vi "Loop_SM.vi"() -> ()   [LabVIEW 2017]
uses:
  ENUM_SM_State.ctl
  ENUM_SM_Action.ctl
  TypeDef/CLUSTER_CMD_WC_Drive.ctl
  TypeDef/ENUM_WC_Drive_DriveMode.ctl
  TypeDef/CLUSTER_Drive_ACT Loop_VBus Data.ctl
  TypeDef/CLUSTER_X and Y.ctl
  TypeDef/CLUSTER_Drive_ACT Loop_Profile Data.ctl
  TypeDef/CLUSTER_Left and Right.ctl
  TypeDef/ENUM_Drive_ACT Loop_Mode.ctl
  TypeDef/CLUSTER_Drive_HW_SRX_Status.ctl
  TypeDef/CLUSTER_4296_SRX_Status.ctl
  TypeDef/CLUSTER_SRX_Status Data.ctl
  TypeDef/CLUSTER_SRX_Encoder Data.ctl
  TypeDef/CLUSTER_SRX_PWM Data.ctl
  TypeDef/CLUSTER_SRX_Analog Data.ctl
  TypeDef/CLUSTER_SRX_Limit Switch Data.ctl
  TypeDef/CLUSTER_SRX_Profile Data.ctl
  TypeDef/CLUST_Targeting Data.ctl
  TypeDef/CLUST_Cube Data.ctl
  TypeDef/CLUST_Road Navigation Data.ctl
  <vilib>/Rock Robotics/WPI/ThirdParty/Sensors/navX/_TypeDefs/FRIC_navX_DeviceNumbersTypeDef.ctl
  _SHARE ALL/Global Share All/Global_STOP.vi
  Globals/Global_CMD_Drive.vi
  Global_ACT Write_Data Out.vi
  Globals/Global_Vision_Data.vi
  Globals/Global_CMD_Gear.vi
  Globals/Global_Drive_Turn_sens.vi
  <vilib>/addons/control/pid/pid.llb/PID (DBL).vi
  Global_SM Write_Data Out.vi
  <vilib>/addons/control/pid/NI_PID_pid.lvlib
  VisionHW Folder/VisionHW.lvlib
panel:
  in  "PID gains Road Follow":T1={"proportional gain (Kc)"=0.01, "integral time (Ti, min)"=0.0, "derivative time (Td, min)"=0.0} {"derivative time (Td, min)" format="%.3f"; "integral time (Ti, min)" format="%.8f"; "proportional gain (Kc)" format="%.8f"}
  in  "PID gains Cube Follow":T1={"proportional gain (Kc)"=0.0015, "integral time (Ti, min)"=0.0, "derivative time (Td, min)"=0.0} {"derivative time (Td, min)" format="%.3f"; "integral time (Ti, min)" format="%.8f"; "proportional gain (Kc)" format="%.8f"}
  in  "Degree allowence":dbl=2.0 format="%#_13g"
  in  "PID gains Lock Angle":T1={"proportional gain (Kc)"=0.01, "integral time (Ti, min)"=0.0, "derivative time (Td, min)"=0.0} {"derivative time (Td, min)" format="%.3f"; "integral time (Ti, min)" format="%.3f"; "proportional gain (Kc)" format="%.8f"}
  in  "Max RPM":dbl=10000.0
  out "Cycle Time (S)":dbl format="%.3g"
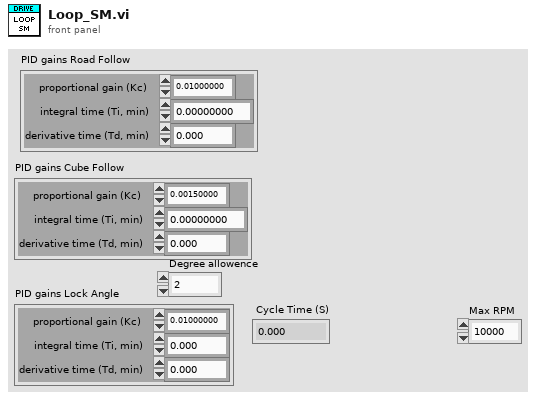
[diagram p1: front panel]
types:
  T1 = cluster{"proportional gain (Kc)":dbl, "integral time (Ti, min)":dbl, "derivative time (Td, min)":dbl}
  T2 = typedef "VisionHW.lvlib/CLUST_Targeting Data.ctl" = cluster{"Cube ":T3, "Road Navigation Data":T4}
  T3 = typedef "VisionHW.lvlib/CLUST_Cube Data.ctl" = cluster{"Height":dbl, "Width":dbl, "Ratio":dbl, "x":i32, "y":i32, "Distance ":i32, "Data Age":dbl}
  T4 = typedef "VisionHW.lvlib/CLUST_Road Navigation Data.ctl" = cluster{"Error":i32, "Data Age":dbl}
  T5 = cluster{"Rollover":dbl, "Yaw":dbl, "Cont Yaw":dbl}
  T6 = typedef "CLUSTER_Drive_HW_SRX_Status.ctl" = cluster{"Rear Left":T7, "Rear Right":T7, "Front Left":T7, "Front Right":T7}
  T7 = typedef "CLUSTER_4296_SRX_Status.ctl" = cluster{"Status":T8, "Encoder":T9, "PWM ":T10, "Analog":T11, "Limit Switches":T12, "Profile":T13}
  T8 = typedef "CLUSTER_SRX_Status Data.ctl" = cluster{"Module Enabled":bool, "Current Profile Slot Select":dbl, "Brake is Enabled":bool, "Applied Throttle":dbl, "Current":dbl, "Battery Voltage":dbl, "Sticky Fault - Under Voltage":bool, "Temperature (C)":dbl, "Sticky Fault - Over Temp":bool, "CAN Error":errorcluster, "Control 5 Is Supported":bool}
  T9 = typedef "CLUSTER_SRX_Encoder Data.ctl" = cluster{"Closed Loop Error":dbl, "Sensor Position":dbl, "Sensor Velocity":dbl, "Encoder Position":dbl, "Encoder Velocity":dbl, "Encoder Index Count":dbl, "Encoder A Pin State":bool, "Encoder B Pin State":bool, "Encoder Index Pin State":bool, "Pos Div 8":bool, "Vel Div 4":bool}
  T10 = typedef "CLUSTER_SRX_PWM Data.ctl" = cluster{"Closed Loop Error":dbl, "Pulse Width Position":i32, "Pulse Width Velocity":i32, "Pulse Width Rise To Rise (us)":i32, "Pulse Width Rise To Fall (us)":i32}
  T11 = typedef "CLUSTER_SRX_Analog Data.ctl" = cluster{"Closed Loop Error":dbl, "Analog In":dbl, "Analog In Velocity":dbl}
  T12 = typedef "CLUSTER_SRX_Limit Switch Data.ctl" = cluster{"Forward Limit Switch Closed":bool, "Reverse Limit Switch Closed":bool, "Sticky Fault - Forward Limit":bool, "Sticky Fault - Reverse Limit":bool, "Sticky Fault - Forward Soft Limit":bool, "Sticky Fault - Reverse Soft Limit":bool}
  T13 = typedef "CLUSTER_SRX_Profile Data.ctl" = cluster{"Mot Prof Active Is Under Run":bool, "Mot Prof Active Has Under Run":bool, "Mot Prof Active Is Last":bool, "Mot Prof Active Velocity Only":bool, "Mot Prof Active Is Valid":bool, "Mot Prof Buffer Is Full":bool, "Mot Prof Active Profile Slot Select":i32, "Mot Prof NextID":i32, "Mot Prof Count":i32, "Mot Prof Active Velocity":dbl, "Mot Prof Active Position":dbl, "Mot Prof Output Enable":i32}
  T14 = typedef "ENUM_Drive_ACT Loop_Mode.ctl" = enum16{"Stop", "Position", "VBus", "Profile"}
  T15 = typedef "CLUSTER_Left and Right.ctl" = cluster{"Left":dbl, "Right":dbl}
  T16 = typedef "CLUSTER_CMD_WC_Drive.ctl" = cluster{"Drive_Mode":T17, "VBus":T18, "Profile":T20, "Zero Drive Encoders":bool, "Set Target Position(IN)":dbl, "Target Angle(Degree)":dbl, "Lock Angle":bool, "Zero YAW":bool, "Follow Cubes":bool, "Follow Road":bool}
  T17 = typedef "ENUM_WC_Drive_DriveMode.ctl" = enum16{"Motion Profile", "CrossLineAuto", "VBus", "Stop"}
  T18 = typedef "CLUSTER_Drive_ACT Loop_VBus Data.ctl" = cluster{"Drive":T19, "Turbo":bool}
  T19 = typedef "CLUSTER_X and Y.ctl" = cluster{"Steer":dbl, "Throtle":dbl}
  T20 = typedef "CLUSTER_Drive_ACT Loop_Profile Data.ctl" = cluster{"Start":bool}
  T21 = typedef "ENUM_SM_Action.ctl" = enum16{"No Action", "Reset Time", "Reset All", "Drive", "Zero YAW", "Shift", "Calculate Sensitivity"}
  T22 = typedef "ENUM_SM_State.ctl" = enum16{"Startup", "VBus", "VBus Lock Angle", "Idle", "Road Follow", "Follow Cube", "Shutdown"}
  T23 = cluster{"Action":T21, "State":T22, "Previous State":T22, "Current Time":timestamp, "Previous Time":timestamp, "Start Time":timestamp, "Target Time (ms)":u32, "Cycle Time(S)":dbl, "CMD_Drive":T16, "VBus Output":T15, "Mode Output":T14, "MQuickStopAccumulator":dbl, "SRX_Status":T6, "Sensitivity":dbl, "NavX Yaw":cluster{"Rollover":dbl, "Yaw":dbl, "Cont Yaw":dbl}, "LockAngle":bool, "Zero YAW":bool, "Target Cube Position (Pixels)":dbl, "Follow Cube":bool, "Follow Road":bool, "Targeting Data":T2, "Gear shift":bool, "Max Sensitivity High Gear":dbl, "Max Sensitivity Low Gear":dbl, "Min Sensitivity High Gear":dbl, "Min Sensitivity Low Gear":dbl}
  T24 = typedef "FRIC_navX_DeviceNumbersTypeDef.ctl" = enum16{"Dev0", "Dev1", "Dev2", "Dev3"}
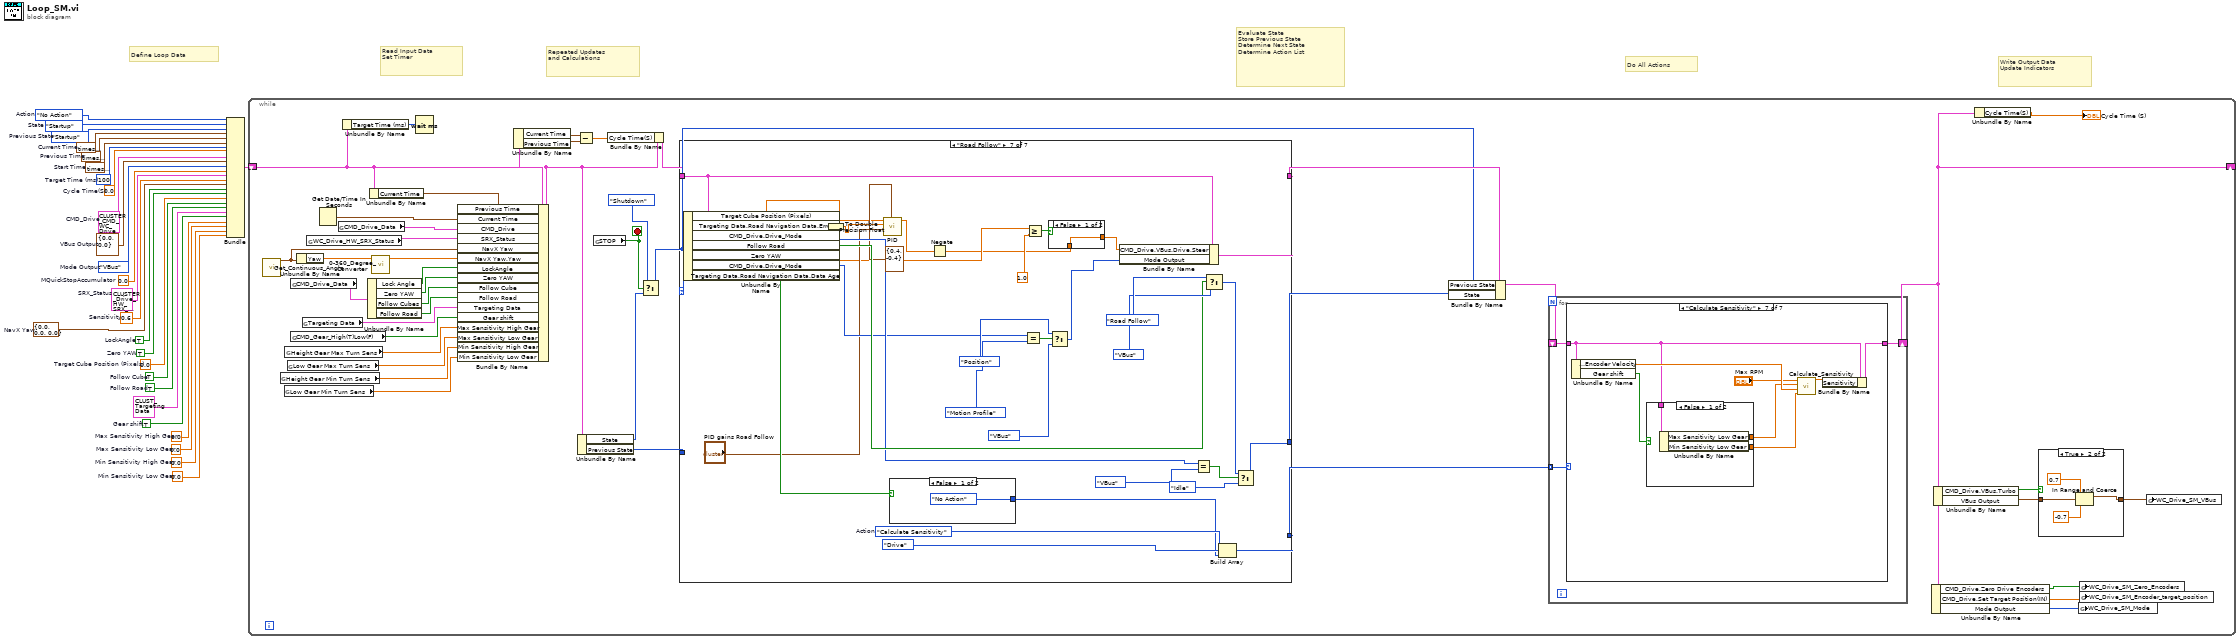
[diagram p0: block diagram]
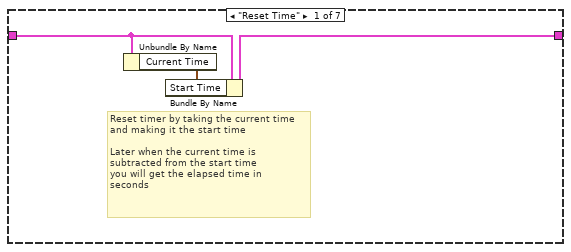
[diagram p3: hidden frame]
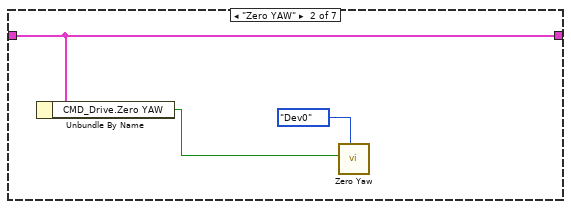
[diagram p4: hidden frame]
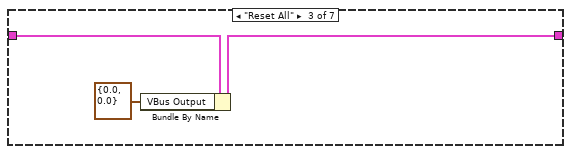
[diagram p5: hidden frame]
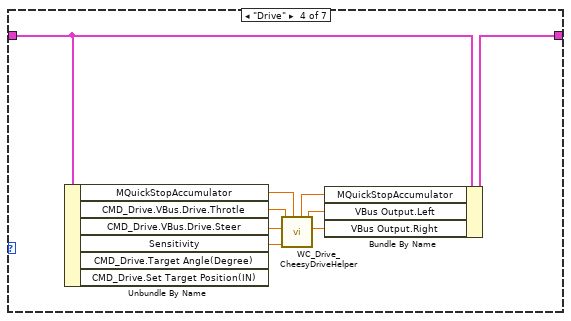
[diagram p6: hidden frame]
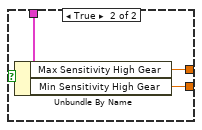
[diagram p9: hidden frame]
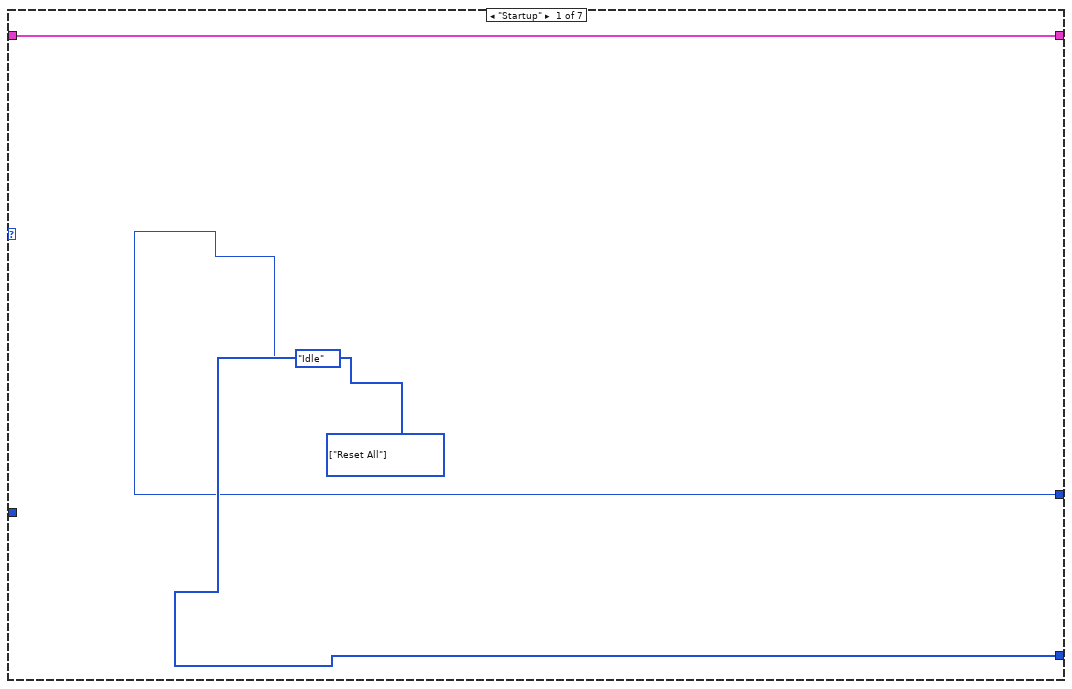
[diagram p10: hidden frame]
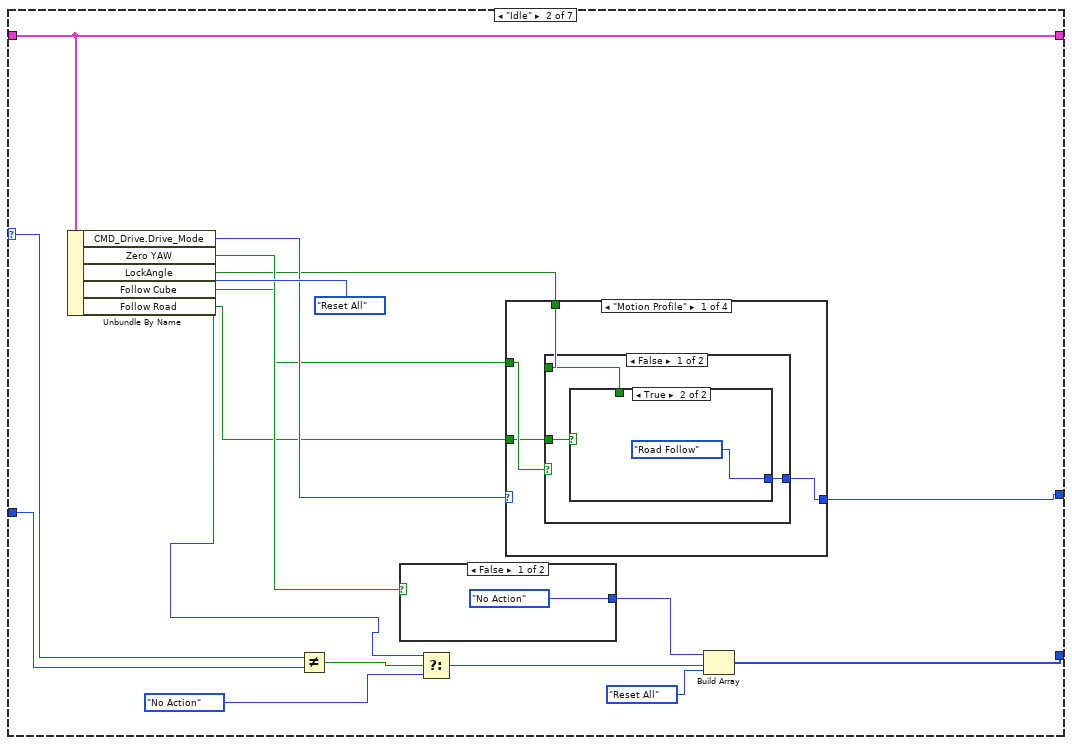
[diagram p11: hidden frame]
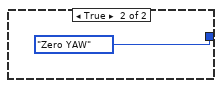
[diagram p12: hidden frame]
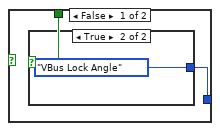
[diagram p13: hidden frame]
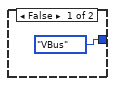
[diagram p14: hidden frame]
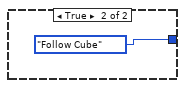
[diagram p15: hidden frame]
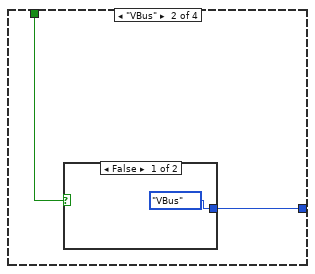
[diagram p16: hidden frame]
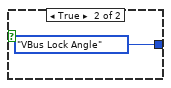
[diagram p17: hidden frame]
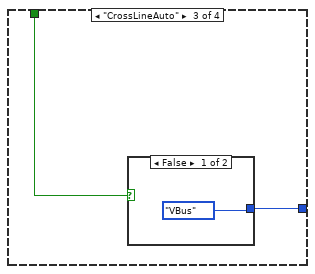
[diagram p18: hidden frame]
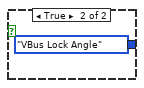
[diagram p19: hidden frame]
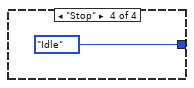
[diagram p20: hidden frame]
diagram:
  w1 = 0.0  # Min Sensitivity Low Gear
  w2 = 0.0  # Min Sensitivity High Gear
  w3 = 0.0  # Max Sensitivity Low Gear
  w4 = 0.0  # Max Sensitivity High Gear
  w5 = TRUE  # Gear shift
  w7 = TRUE  # Follow Road
  w8 = TRUE  # Follow Cube
  w9 = 0.0  # Target Cube Position (Pixels)
  w10 = TRUE  # Zero YAW
  w11 = TRUE  # LockAngle
  w12 = T5 {"Rollover"=0.0, "Yaw"=0.0, "Cont Yaw"=0.0}  # NavX Yaw
  w13 = 0.6  # Sensitivity
  w14 = T6 {"Rear Left"={"Status"={"Module Enabled"=FALSE, "Current Profile Slot Select"=0.0, "Brake is Enabled"=TRUE, "Applied Throttle"=0.0, "Current"=0.0, "Battery Voltage"=12.450000000000001, "Sticky Fault - Under Voltage"=TRUE, "Temperature (C)"=30.645161290322577, "Sticky Fault - Over Temp"=FALSE, "CAN Error"={"status"=FALSE, "code"=0, "source"=""}, "Control 5 Is Supported"=TRUE}, "Encoder"={"Closed Loop Error"=0.0, "Sensor Position"=-847.859619140625, "Sensor Velocity"=0.0, "Encoder Position"=-3472833.0, "Encoder Velocity"=0.0, "Encoder Index Count"=-9452.0, "Encoder A Pin State"=FALSE, "Encoder B Pin State"=FALSE, "Encoder Index Pin State"=FALSE, "Pos Div 8"=FALSE, "Vel Div 4"=FALSE}, "PWM "={"Closed Loop Error"=0.0, "Pulse Width Position"=-3472224, "Pulse Width Velocity"=0, "Pulse Width Rise To Rise (us)"=4187, "Pulse Width Rise To Fall (us)"=1210}, "Analog"={"Closed Loop Error"=0.0, "Analog In"=105.0, "Analog In Velocity"=0.0}, "Limit Switches"={"Forward Limit Switch Closed"=FALSE, "Reverse Limit Switch Closed"=FALSE, "Sticky Fault - Forward Limit"=FALSE, "Sticky Fault - Reverse Limit"=TRUE, "Sticky Fault - Forward Soft Limit"=FALSE, "Sticky Fault - Reverse Soft Limit"=FALSE}, "Profile"={"Mot Prof Active Is Under Run"=FALSE, "Mot Prof Active Has Under Run"=FALSE, "Mot Prof Active Is Last"=FALSE, "Mot Prof Active Velocity Only"=FALSE, "Mot Prof Active Is Valid"=FALSE, "Mot Prof Buffer Is Full"=FALSE, "Mot Prof Active Profile Slot Select"=0, "Mot Prof NextID"=0, "Mot Prof Count"=0, "Mot Prof Active Velocity"=0.0, "Mot Prof Active Position"=0.0, "Mot Prof Output Enable"=0}}, "Rear Right"={"Status"={"Module Enabled"=FALSE, "Current Profile Slot Select"=0.0, "Brake is Enabled"=TRUE, "Applied Throttle"=0.0, "Current"=0.125, "Battery Voltage"=12.4, "Sticky Fault - Under Voltage"=TRUE, "Temperature (C)"=27.41935483870968, "Sticky Fault - Over Temp"=FALSE, "CAN Error"={"status"=FALSE, "code"=0, "source"=""}, "Control 5 Is Supported"=TRUE}, "Encoder"={"Closed Loop Error"=0.0, "Sensor Position"=-228.95263671875, "Sensor Velocity"=0.0, "Encoder Position"=937790.0, "Encoder Velocity"=0.0, "Encoder Index Count"=2928.0, "Encoder A Pin State"=FALSE, "Encoder B Pin State"=TRUE, "Encoder Index Pin State"=TRUE, "Pos Div 8"=FALSE, "Vel Div 4"=FALSE}, "PWM "={"Closed Loop Error"=0.0, "Pulse Width Position"=937817, "Pulse Width Velocity"=0, "Pulse Width Rise To Rise (us)"=4128, "Pulse Width Rise To Fall (us)"=3960}, "Analog"={"Closed Loop Error"=0.0, "Analog In"=103.0, "Analog In Velocity"=0.0}, "Limit Switches"={"Forward Limit Switch Closed"=FALSE, "Reverse Limit Switch Closed"=FALSE, "Sticky Fault - Forward Limit"=FALSE, "Sticky Fault - Reverse Limit"=FALSE, "Sticky Fault - Forward Soft Limit"=FALSE, "Sticky Fault - Reverse Soft Limit"=FALSE}, "Profile"={"Mot Prof Active Is Under Run"=FALSE, "Mot Prof Active Has Under Run"=FALSE, "Mot Prof Active Is Last"=FALSE, "Mot Prof Active Velocity Only"=FALSE, "Mot Prof Active Is Valid"=FALSE, "Mot Prof Buffer Is Full"=FALSE, "Mot Prof Active Profile Slot Select"=0, "Mot Prof NextID"=0, "Mot Prof Count"=0, "Mot Prof Active Velocity"=0.0, "Mot Prof Active Position"=0.0, "Mot Prof Output Enable"=0}}, "Front Left"={"Status"={"Module Enabled"=FALSE, "Current Profile Slot Select"=0.0, "Brake is Enabled"=TRUE, "Applied Throttle"=0.0, "Current"=0.0, "Battery Voltage"=12.4, "Sticky Fault - Under Voltage"=TRUE, "Temperature (C)"=28.709677419354833, "Sticky Fault - Over Temp"=FALSE, "CAN Error"={"status"=FALSE, "code"=0, "source"=""}, "Control 5 Is Supported"=TRUE}, "Encoder"={"Closed Loop Error"=0.0, "Sensor Position"=0.0, "Sensor Velocity"=0.0, "Encoder Position"=0.0, "Encoder Velocity"=0.0, "Encoder Index Count"=0.0, "Encoder A Pin State"=TRUE, "Encoder B Pin State"=TRUE, "Encoder Index Pin State"=TRUE, "Pos Div 8"=FALSE, "Vel Div 4"=FALSE}, "PWM "={"Closed Loop Error"=0.0, "Pulse Width Position"=0, "Pulse Width Velocity"=0, "Pulse Width Rise To Rise (us)"=0, "Pulse Width Rise To Fall (us)"=0}, "Analog"={"Closed Loop Error"=0.0, "Analog In"=105.0, "Analog In Velocity"=0.0}, "Limit Switches"={"Forward Limit Switch Closed"=FALSE, "Reverse Limit Switch Closed"=FALSE, "Sticky Fault - Forward Limit"=FALSE, "Sticky Fault - Reverse Limit"=FALSE, "Sticky Fault - Forward Soft Limit"=FALSE, "Sticky Fault - Reverse Soft Limit"=FALSE}, "Profile"={"Mot Prof Active Is Under Run"=FALSE, "Mot Prof Active Has Under Run"=FALSE, "Mot Prof Active Is Last"=FALSE, "Mot Prof Active Velocity Only"=FALSE, "Mot Prof Active Is Valid"=FALSE, "Mot Prof Buffer Is Full"=FALSE, "Mot Prof Active Profile Slot Select"=0, "Mot Prof NextID"=0, "Mot Prof Count"=0, "Mot Prof Active Velocity"=0.0, "Mot Prof Active Position"=0.0, "Mot Prof Output Enable"=0}}, "Front Right"={"Status"={"Module Enabled"=FALSE, "Current Profile Slot Select"=0.0, "Brake is Enabled"=TRUE, "Applied Throttle"=0.0, "Current"=0.0, "Battery Voltage"=12.35, "Sticky Fault - Under Voltage"=TRUE, "Temperature (C)"=26.77419354838709, "Sticky Fault - Over Temp"=FALSE, "CAN Error"={"status"=FALSE, "code"=0, "source"=""}, "Control 5 Is Supported"=TRUE}, "Encoder"={"Closed Loop Error"=0.0, "Sensor Position"=0.0, "Sensor Velocity"=0.0, "Encoder Position"=0.0, "Encoder Velocity"=0.0, "Encoder Index Count"=0.0, "Encoder A Pin State"=TRUE, "Encoder B Pin State"=TRUE, "Encoder Index Pin State"=TRUE, "Pos Div 8"=FALSE, "Vel Div 4"=FALSE}, "PWM "={"Closed Loop Error"=0.0, "Pulse Width Position"=0, "Pulse Width Velocity"=0, "Pulse Width Rise To Rise (us)"=0, "Pulse Width Rise To Fall (us)"=0}, "Analog"={"Closed Loop Error"=0.0, "Analog In"=102.0, "Analog In Velocity"=0.0}, "Limit Switches"={"Forward Limit Switch Closed"=FALSE, "Reverse Limit Switch Closed"=FALSE, "Sticky Fault - Forward Limit"=FALSE, "Sticky Fault - Reverse Limit"=TRUE, "Sticky Fault - Forward Soft Limit"=FALSE, "Sticky Fault - Reverse Soft Limit"=FALSE}, "Profile"={"Mot Prof Active Is Under Run"=FALSE, "Mot Prof Active Has Under Run"=FALSE, "Mot Prof Active Is Last"=FALSE, "Mot Prof Active Velocity Only"=FALSE, "Mot Prof Active Is Valid"=FALSE, "Mot Prof Buffer Is Full"=FALSE, "Mot Prof Active Profile Slot Select"=0, "Mot Prof NextID"=0, "Mot Prof Count"=0, "Mot Prof Active Velocity"=0.0, "Mot Prof Active Position"=0.0, "Mot Prof Output Enable"=0}}}  # SRX_Status
  w15 = 0.0  # MQuickStopAccumulator
  w16 = ENUM_Drive_ACT_Loop_Mode."VBus"  # Mode Output
  w17 = T15 {"Left"=0.0, "Right"=0.0}  # VBus Output
  w18 = T16 {"Drive_Mode"=enum."Motion Profile", "VBus"={"Drive"={"Steer"=0.0, "Throtle"=0.0}, "Turbo"=FALSE}, "Profile"={"Start"=FALSE}, "Zero Drive Encoders"=FALSE, "Set Target Position(IN)"=0.0, "Target Angle(Degree)"=0.0, "Lock Angle"=FALSE, "Zero YAW"=FALSE, "Follow Cubes"=FALSE, "Follow Road"=FALSE}  # CMD_Drive
  w19 = ENUM_SM_Action."No Action"  # Action
  w20 = 0.0  # Cycle Time(S)
  w21 = ENUM_SM_State."Startup"  # Previous State
  w22 = timestamp(0 s since 1904-01-01)  # Previous Time
  w23 = u32 100  # Target Time (ms)
  w24 = timestamp(0 s since 1904-01-01)  # Start Time
  w25 = timestamp(0 s since 1904-01-01)  # Current Time
  w26 = ENUM_SM_State."Startup"  # State
  # "Define Loop Data"
  # "Repeated Updates\nand Calculations"
  # "Read Input Data\nSet Timer"
  # "Evaluate State\nStore Previous State\nDetermine Next State\nDetermine Action List"
  # "Do All Actions"
  # "Write Output Data\nUpdate Indicators"
  n1 = Bundle("Action"=w19, "State"=w26, "Previous State"=w21, "Current Time"=w25, "Previous Time"=w22, "Start Time"=w24, "Target Time (ms)"=w23, "Cycle Time(S)"=w20, "CMD_Drive"=w18, "VBus Output"=w17, "Mode Output"=w16, "MQuickStopAccumulator"=w15, "SRX_Status"=w14, "Sensitivity"=w13, "NavX Yaw"=w12, "LockAngle"=w11, "Zero YAW"=w10, "Target Cube Position (Pixels)"=w9, "Follow Cube"=w8, "Follow Road"=w7, "Targeting Data"=T2 {"Cube "={"Height"=0.0, "Width"=0.0, "Ratio"=0.0, "x"=0, "y"=0, "Distance "=0, "Data Age"=0.0}, "Road Navigation Data"={"Error"=0, "Data Age"=0.0}}, "Gear shift"=w5, "Max Sensitivity High Gear"=w4, "Max Sensitivity Low Gear"=w3, "Min Sensitivity High Gear"=w2, "Min Sensitivity Low Gear"=w1) -> (w27:T23)  [unwired: 1 in]
  n2 = while {
    shift-right: [w49] -> _
    shift-left: w27 -> [w60]
    stop <- w65 stop-if-true
    n3 = call <vilib>:"Get_Continuous_Angle.vi"() -> ("Continuous Angle"=w45:T5)  [unwired: 11 in]
    n4 = global read "Global_Drive_Turn_sens.vi" "Height Gear Min Turn Sens"() -> (w29:dbl)
    n5 = global read "Global_Drive_Turn_sens.vi" "Low Gear Min Turn Sens"() -> (w28:dbl)
    n6 = global read "Global_Drive_Turn_sens.vi" "Height Gear Max Turn Sens"() -> (w31:dbl)
    n7 = global read "Global_Drive_Turn_sens.vi" "Low Gear Max Turn Sens"() -> (w30:dbl)
    n8 = global read "Global_CMD_Drive.vi" "CMD_Drive_Data"() -> (w40:T16)
    n9 = global read "Global_CMD_Gear.vi" "CMD_Gear_High(T)Low(F)"() -> (w32:bool)
    n10 = Unbundle By Name(w45) -> ("Yaw"=w44:dbl)
    n11 = global read "Global_Vision_Data.vi" "Targeting Data"() -> (w33:T2)
    n12 = global read "Global_ACT Write_Data Out.vi" "WC_Drive_HW_SRX_Status"() -> (w46:T6)
    n13 = Get Date/Time In Seconds() -> (seconds since 1Jan1904=w69:timestamp)
    n14 = global read "Global_CMD_Drive.vi" "CMD_Drive_Data"() -> (w50:T16)
    n15 = Unbundle By Name(w60) -> ("Target Time (ms)"=w62:u32)
    n16 = Unbundle By Name(w40) -> ("Lock Angle"=w39:bool, "Zero YAW"=w38:bool, "Follow Cubes"=w35:bool, "Follow Road"=w34:bool)
    n17 = Unbundle By Name(w60) -> ("Current Time"=w61:timestamp)
    n18 = call "0-360_Degree_Converter.vi"("Yaw in"=w44) -> ("Yaw out"=w41:dbl)  [unwired: 10 in]
    n19 = Wait (ms)(milliseconds to wait=w62) -> ()  [unwired: 1 out]
    n20 = Bundle By Name(cluster=w60, "Previous Time"=w61, "Current Time"=w69, "CMD_Drive"=w50, "SRX_Status"=w46, "NavX Yaw"=w45, "NavX Yaw.Yaw"=w41, "LockAngle"=w39, "Zero YAW"=w38, "Follow Cube"=w35, "Follow Road"=w34, "Targeting Data"=w33, "Gear shift"=w32, "Max Sensitivity High Gear"=w31, "Max Sensitivity Low Gear"=w30, "Min Sensitivity High Gear"=w29, "Min Sensitivity Low Gear"=w28) -> (w42:T23)
    n21 = Unbundle By Name(w42) -> ("Current Time"=w55:timestamp, "Previous Time"=w56:timestamp)
    n22 = Subtract(x=w55, y=w56) -> (x-y=w53:dbl)
    n23 = Unbundle By Name(w42) -> ("State"=w63:T22, "Previous State"=w59:T22)
    n24 = global read "Global_STOP.vi" "STOP"() -> (w65:bool)
    n25 = Bundle By Name(cluster=w42, "Cycle Time(S)"=w53) -> (w54:T23)
    n26 = Select(t=ENUM_SM_State."Shutdown" ("State"), s=w65, f=w63) -> (s? t:f=w58:T22)
    n27 = case shown="\"Road Follow\"" w58 {
      selector: w58 -> [_ w124 _ _ _ _ _]
      tunnel: w54 -> [w114 w130 w159 w188 w213 w248 w285]
      tunnel: [w114 w130 w158 w188 w217 w252 w289] -> w67
      tunnel: [ENUM_SM_State."Idle" ("State") w121 w178 ENUM_SM_State."Shutdown" ("State") w205 w241 w278] -> w66
      tunnel: [w113 w125 w174 w186 w214 w249 w286] -> w52
      tunnel: w59 -> [_ w123 _ _ _ _ _]
      frame "Startup" {
        w113 = T21[] [enum."Reset All"] items=["No Action", "Reset Time", "Reset All", "Drive", "Zero YAW", "Shift", "Calculate Sensitivity"] ("Actions")
      }
      frame "Idle" {
        n28 = Unbundle By Name(w130) -> ("CMD_Drive.Drive_Mode"=w122:T17, "Zero YAW"=w119:bool, "LockAngle"=w118:bool, "Follow Cube"=w116:bool, "Follow Road"=w115:bool)
        n29 = Not Equal?(x=w124, y=w123) -> (x != y?=w129:bool)
        n30 = case shown="False" w119 {
          tunnel: [ENUM_SM_Action."No Action" ("element") ENUM_SM_Action."Zero YAW" ("element")] -> w120
          frame False {
          }
          frame True {
          }
        }
        n31 = Select(t=ENUM_SM_Action."Reset All" ("Action"), s=w129, f=ENUM_SM_Action."No Action" ("Action")) -> (s? t:f=w128:T21)
        n32 = case shown="\"Motion Profile\"" w122 {
          tunnel: [w136 w147 w151 ENUM_SM_State."Idle" ("State")] -> w121
          tunnel: w118 -> [w135 w146 w150 _]
          tunnel: w116 -> [w134 _ _ _]
          tunnel: w115 -> [w133 _ _ _]
          frame "Motion Profile" {
            n33 = case shown="False" w134 {
              tunnel: [w139 ENUM_SM_State."Follow Cube" ("State")] -> w136
              tunnel: w135 -> [w138 _]
              tunnel: w133 -> [w137 _]
              frame False {
                n34 = case shown="True" w137 {
                  tunnel: [w141 ENUM_SM_State."Road Follow" ("State")] -> w139
                  tunnel: w138 -> [w140 _]
                  frame False {
                    n35 = case shown="True" w140 {
                      tunnel: [ENUM_SM_State."VBus" ("State") ENUM_SM_State."VBus Lock Angle" ("State")] -> w141
                      frame False {
                      }
                      frame True {
                      }
                    }
                  }
                  frame True {
                  }
                }
              }
              frame True {
              }
            }
          }
          frame "VBus" {
            n36 = case shown="False" w146 {
              tunnel: [ENUM_SM_State."VBus" ("State") ENUM_SM_State."VBus Lock Angle" ("State")] -> w147
              frame False {
              }
              frame True {
              }
            }
          }
          frame "CrossLineAuto" {
            n37 = case shown="False" w150 {
              tunnel: [ENUM_SM_State."VBus" ("State") ENUM_SM_State."VBus Lock Angle" ("State")] -> w151
              frame False {
              }
              frame True {
              }
            }
          }
          frame "Stop" {
          }
        }
        n38 = Build Array(w120, w128, ENUM_SM_Action."Reset All" ("element")) -> (w125:T21[])
      }
      frame "VBus" {
        w175 = ENUM_SM_Action."Calculate Sensitivity"  # Action
        n39 = Unbundle By Name(w159) -> ("CMD_Drive.Drive_Mode"=w177:T17, "LockAngle"=w169:bool, "Zero YAW"=w166:bool, "CMD_Drive.Drive_Mode"=w162:T17, "Follow Cube"=w156:bool, "Follow Road"=w155:bool)
        n40 = case shown="True" w155 {
          tunnel: [w180 ENUM_SM_State."Road Follow" ("State")] -> w167
          tunnel: w156 -> [w179 _]
          frame False {
            n41 = case shown="False" w179 {
              tunnel: [ENUM_SM_State."VBus" ("State") ENUM_SM_State."Follow Cube" ("State")] -> w180
              frame False {
              }
              frame True {
              }
            }
          }
          frame True {
          }
        }
        n42 = case shown="False" w166 {
          tunnel: [ENUM_SM_Action."No Action" ("element") ENUM_SM_Action."Zero YAW" ("element")] -> w165
          frame False {
          }
          frame True {
          }
        }
        n43 = Equal?(x=w162, y=ENUM_WC_Drive_DriveMode."Motion Profile" ("CMD_Drive.Drive_Mode")) -> (x = y?=w164:bool)
        n44 = Select(t=ENUM_Drive_ACT_Loop_Mode."Position" ("WC_Drive_SM_Mode"), s=w164, f=ENUM_Drive_ACT_Loop_Mode."VBus" ("WC_Drive_SM_Mode")) -> (s? t:f=w157:T14)
        n45 = Equal?(x=w177, y=ENUM_WC_Drive_DriveMode."VBus" ("CMD_Drive_Mode")) -> (x = y?=w176:bool)
        n46 = Select(t=ENUM_SM_State."VBus Lock Angle" ("State"), s=w169, f=w167) -> (s? t:f=w170:T22)
        n47 = Bundle By Name(cluster=w159, "Mode Output"=w157) -> (w158:T23)
        n48 = Build Array(w175, ENUM_SM_Action."Drive" ("element"), w165) -> (w174:T21[])
        n49 = Select(t=w170, s=w176, f=ENUM_SM_State."Idle" ("State")) -> (s? t:f=w178:T22)
      }
      frame "Shutdown" {
        w186 = T21[] [enum."Reset All"] items=["No Action", "Reset Time", "Reset All", "Drive", "Zero YAW", "Shift", "Calculate Sensitivity"] ("Actions")
      }
      frame "VBus Lock Angle" {
        w216 = ENUM_SM_Action."Calculate Sensitivity"  # Action
        n50 = Unbundle By Name(w213) -> ("CMD_Drive.Target Angle(Degree)"=w196:dbl, "NavX Yaw.Yaw"=w199:dbl, "CMD_Drive.Drive_Mode"=w203:T17, "LockAngle"=w204:bool, "Zero YAW"=w197:bool, "CMD_Drive.Drive_Mode"=w191:T17)
        n51 = call-poly <vilib>:"PID.vi"("output range"=cluster{"output high":dbl, "output low":dbl} {"output high"=1.0, "output low"=-1.0}, "PID gains"="PID gains Lock Angle", "process variable"=w199, "setpoint"=w196) -> ("output"=w200:dbl)  [unwired: 6 in, 1 out]
        n52 = case shown="False" w197 {
          tunnel: [ENUM_SM_Action."No Action" ("element") ENUM_SM_Action."Zero YAW" ("element")] -> w198
          frame False {
          }
          frame True {
          }
        }
        n53 = call "Steering_converter.vi"("Yaw"=w199, "setpoint"=w196, "output"=w200, "Degree allowence"="Degree allowence") -> ("Steer"=w201:dbl)  [unwired: 7 in]
        n54 = Equal?(x=w191, y=ENUM_WC_Drive_DriveMode."Motion Profile" ("CMD_Drive.Drive_Mode")) -> (x = y?=w195:bool)
        n55 = Select(t=ENUM_Drive_ACT_Loop_Mode."Position" ("WC_Drive_SM_Mode"), s=w195, f=ENUM_Drive_ACT_Loop_Mode."VBus" ("WC_Drive_SM_Mode")) -> (s? t:f=w190:T14)
        n56 = Bundle By Name(cluster=w213, "CMD_Drive.VBus.Drive.Steer"=w201, "Mode Output"=w190) -> (w217:T23)
        n57 = Equal?(x=w203, y=ENUM_WC_Drive_DriveMode."VBus" ("CMD_Drive_Mode")) -> (x = y?=w211:bool)
        n58 = Select(t=ENUM_SM_State."VBus Lock Angle" ("State"), s=w204, f=ENUM_SM_State."VBus" ("State")) -> (s? t:f=w208:T22)
        n59 = Build Array(w216, ENUM_SM_Action."Drive" ("element"), w198) -> (w214:T21[])
        n60 = Select(t=w208, s=w211, f=ENUM_SM_State."Idle" ("State")) -> (s? t:f=w205:T22)
      }
      frame "Follow Cube" {
        w251 = ENUM_SM_Action."Calculate Sensitivity"  # Action
        n61 = Unbundle By Name(w248) -> ("Target Cube Position (Pixels)"=w235:dbl, "Targeting Data.Cube.x"=w227:i32, "CMD_Drive.Drive_Mode"=w239:T17, "Follow Cube"=w240:bool, "Zero YAW"=w236:bool, "CMD_Drive.Drive_Mode"=w230:T17, "Targeting Data.Cube.Data Age"=w225:dbl)
        n62 = To Double Precision Float(number=w227) -> (double precision float=w222:dbl)
        n63 = call-poly <vilib>:"PID.vi"("output range"=cluster{"output high":dbl, "output low":dbl} {"output high"=0.4, "output low"=-0.4}, "PID gains"="PID gains Cube Follow", "process variable"=w222, "setpoint"=w235) -> ("output"=w221:dbl)  [unwired: 6 in, 1 out]
        n64 = case shown="False" w236 {
          tunnel: [ENUM_SM_Action."No Action" ("element") ENUM_SM_Action."Zero YAW" ("element")] -> w237
          frame False {
          }
          frame True {
          }
        }
        n65 = Negate(x=w221) -> (-x=w220:dbl)
        n66 = Equal?(x=w230, y=ENUM_WC_Drive_DriveMode."Motion Profile" ("CMD_Drive.Drive_Mode")) -> (x = y?=w234:bool)
        n67 = Greater Or Equal?(x=w225, y=1.0) -> (x >= y?=w226:bool)
        n68 = case shown="False" w226 {
          tunnel: [w253 0.0 ("CMD_Drive.VBus.Drive.Steer")] -> w223
          tunnel: w220 -> [w253 _]
          frame False {
          }
          frame True {
          }
        }
        n69 = Select(t=ENUM_Drive_ACT_Loop_Mode."Position" ("WC_Drive_SM_Mode"), s=w234, f=ENUM_Drive_ACT_Loop_Mode."VBus" ("WC_Drive_SM_Mode")) -> (s? t:f=w229:T14)
        n70 = Bundle By Name(cluster=w248, "CMD_Drive.VBus.Drive.Steer"=w223, "Mode Output"=w229) -> (w252:T23)
        n71 = Equal?(x=w239, y=ENUM_WC_Drive_DriveMode."VBus" ("CMD_Drive_Mode")) -> (x = y?=w247:bool)
        n72 = Select(t=ENUM_SM_State."Follow Cube" ("State"), s=w240, f=ENUM_SM_State."VBus" ("State")) -> (s? t:f=w244:T22)
        n73 = Build Array(w251, ENUM_SM_Action."Drive" ("element"), w237) -> (w249:T21[])
        n74 = Select(t=w244, s=w247, f=ENUM_SM_State."Idle" ("State")) -> (s? t:f=w241:T22)
      }
      frame "Road Follow" {
        w288 = ENUM_SM_Action."Calculate Sensitivity"  # Action
        n75 = Unbundle By Name(w285) -> ("Target Cube Position (Pixels)"=w272:dbl, "Targeting Data.Road Navigation Data.Error"=w264:i32, "CMD_Drive.Drive_Mode"=w276:T17, "Follow Road"=w277:bool, "Zero YAW"=w273:bool, "CMD_Drive.Drive_Mode"=w267:T17, "Targeting Data.Road Navigation Data.Data Age"=w262:dbl)
        n76 = To Double Precision Float(number=w264) -> (double precision float=w259:dbl)
        n77 = call-poly <vilib>:"PID.vi"("output range"=cluster{"output high":dbl, "output low":dbl} {"output high"=0.4, "output low"=-0.4}, "PID gains"="PID gains Road Follow", "process variable"=w259, "setpoint"=w272) -> ("output"=w258:dbl)  [unwired: 6 in, 1 out]
        n78 = case shown="False" w273 {
          tunnel: [ENUM_SM_Action."No Action" ("element") ENUM_SM_Action."Zero YAW" ("element")] -> w274
          frame False {
          }
          frame True {
          }
        }
        n79 = Negate(x=w258) -> (-x=w257:dbl)
        n80 = Equal?(x=w267, y=ENUM_WC_Drive_DriveMode."Motion Profile" ("CMD_Drive.Drive_Mode")) -> (x = y?=w271:bool)
        n81 = Greater Or Equal?(x=w262, y=1.0) -> (x >= y?=w263:bool)
        n82 = case shown="False" w263 {
          tunnel: [w290 0.0 ("CMD_Drive.VBus.Drive.Steer")] -> w260
          tunnel: w257 -> [w290 _]
          frame False {
          }
          frame True {
          }
        }
        n83 = Select(t=ENUM_Drive_ACT_Loop_Mode."Position" ("WC_Drive_SM_Mode"), s=w271, f=ENUM_Drive_ACT_Loop_Mode."VBus" ("WC_Drive_SM_Mode")) -> (s? t:f=w266:T14)
        n84 = Bundle By Name(cluster=w285, "CMD_Drive.VBus.Drive.Steer"=w260, "Mode Output"=w266) -> (w289:T23)
        n85 = Equal?(x=w276, y=ENUM_WC_Drive_DriveMode."VBus" ("CMD_Drive_Mode")) -> (x = y?=w284:bool)
        n86 = Select(t=ENUM_SM_State."Road Follow" ("State"), s=w277, f=ENUM_SM_State."VBus" ("State")) -> (s? t:f=w281:T22)
        n87 = Build Array(w288, ENUM_SM_Action."Drive" ("element"), w274) -> (w286:T21[])
        n88 = Select(t=w281, s=w284, f=ENUM_SM_State."Idle" ("State")) -> (s? t:f=w278:T22)
      }
    }
    n89 = Bundle By Name(cluster=w67, "Previous State"=w58, "State"=w66) -> (w68:T23)
    n90 = for {
      tunnel: w52 -> [w77] mode=indexing
      shift-right: [w76] -> w49
      shift-left: w68 -> [w75]
      n91 = case shown="\"Calculate Sensitivity\"" w77 {
        tunnel: w75 -> [w80 w82 w86 w95 w96 w97 w100]
        tunnel: [w79 w82 w85 w94 w96 w97 w105] -> w76
        frame "Reset Time" {
          # "Reset timer by taking the current time\nand making it the start time\n\nLater when the current time is \nsubtracted from the start time\nyou will get the elapsed time in \nseconds"
          n92 = Unbundle By Name(w80) -> ("Current Time"=w78:timestamp)
          n93 = Bundle By Name(cluster=w80, "Start Time"=w78) -> (w79:T23)
        }
        frame "Zero YAW" {
          n94 = Unbundle By Name(w82) -> ("CMD_Drive.Zero YAW"=w81:bool)
          n95 = call <vilib>:"Zero Yaw.vi"("Device Number"=FRIC_navX_DeviceNumbersTypeDef."Dev0", "Zero"=w81) -> ()  [unwired: 10 in]
        }
        frame "Reset All" {
          n96 = Bundle By Name(cluster=w86, "VBus Output"=T15 {"Left"=0.0, "Right"=0.0}) -> (w85:T23)
        }
        frame "Drive" {
          n97 = Unbundle By Name(w95) -> ("MQuickStopAccumulator"=w92:dbl, "CMD_Drive.VBus.Drive.Throtle"=w91:dbl, "CMD_Drive.VBus.Drive.Steer"=w90:dbl, "Sensitivity"=w89:dbl)  [unwired: 2 out]
          n98 = call "WC_Drive_CheesyDriveHelper.vi"("MQuickStopAccumulator"=w92, "KTurnSensitivity"=w89, "Steer"=w90, "Throttle"=w91) -> ("RightPwm Out"=w87:dbl, "LeftPwm Out"=w88:dbl, "MQuickStopAccumulator Out"=w93:dbl)  [unwired: 5 in]
          n99 = Bundle By Name(cluster=w95, "MQuickStopAccumulator"=w93, "VBus Output.Left"=w88, "VBus Output.Right"=w87) -> (w94:T23)
        }
        frame "No Action" {
        }
        frame "Shift" {
        }
        frame "Calculate Sensitivity" {
          n100 = Unbundle By Name(w100) -> ("SRX_Status.Rear Right.Encoder.Encoder Velocity"=w103:dbl, "Gear shift"=w101:bool)
          n101 = case shown="False" w101 {
            tunnel: w100 -> [w108 w111]
            tunnel: [w107 w110] -> w99
            tunnel: [w106 w109] -> w98
            frame False {
              n102 = Unbundle By Name(w108) -> ("Max Sensitivity Low Gear"=w107:dbl, "Min Sensitivity Low Gear"=w106:dbl)
            }
            frame True {
              n103 = Unbundle By Name(w111) -> ("Max Sensitivity High Gear"=w110:dbl, "Min Sensitivity High Gear"=w109:dbl)
            }
          }
          n104 = call "Calculate_Sensitivity.vi"("Min Sensitivity"=w98, "Current RPM"=w103, "Max Sensitivity"=w99, "Max RPM"="Max RPM") -> ("Sensitivity"=w104:dbl)  [unwired: 7 in]
          n105 = Bundle By Name(cluster=w100, "Sensitivity"=w104) -> (w105:T23)
        }
      }
    }
    n106 = Unbundle By Name(w49) -> ("CMD_Drive.Zero Drive Encoders"=w36:bool, "CMD_Drive.Set Target Position(IN)"=w37:dbl, "Mode Output"=w43:T14)
    n107 = Unbundle By Name(w49) -> ("CMD_Drive.VBus.Turbo"=w47:bool, "VBus Output"=w51:T15)
    n108 = Unbundle By Name(w49) -> ("Cycle Time(S)"=→"Cycle Time (S)":dbl)
    n109 = case shown="True" w47 {
      tunnel: w51 -> [w70 w74]
      tunnel: [w70 w71] -> w48
      frame False {
      }
      frame True {
        n110 = In Range and Coerce(upper limit=0.7, x=w74, lower limit=-0.7) -> (coerced(x)=w71:T15)  [unwired: 1 out]
      }
    }
    n111 = global write "Global_SM Write_Data Out.vi" "WC_Drive_SM_Mode"(w43) -> ()
    n112 = global write "Global_SM Write_Data Out.vi" "WC_Drive_SM_Zero_Encoders"(w36) -> ()
    n113 = global write "Global_SM Write_Data Out.vi" "WC_Drive_SM_Encoder_target_position"(w37) -> ()
    n114 = global write "Global_SM Write_Data Out.vi" "WC_Drive_SM_VBus"(w48) -> ()
  }
